vi "GetRingText.vi"(8 "error in (no error)":errorcluster, 11 "RingItem in":refnum<class "RingItem.lvclass">) -> (0 "error out":errorcluster, 2 "ring text":string, 3 "RingItem out":refnum<class "RingItem.lvclass">)   [LabVIEW 2009, in "NavScreen.lvlib" / "RingItem.lvclass"]
uses:
  RingItem.lvclass
  RingItem.lvclass/RingItem.ctl
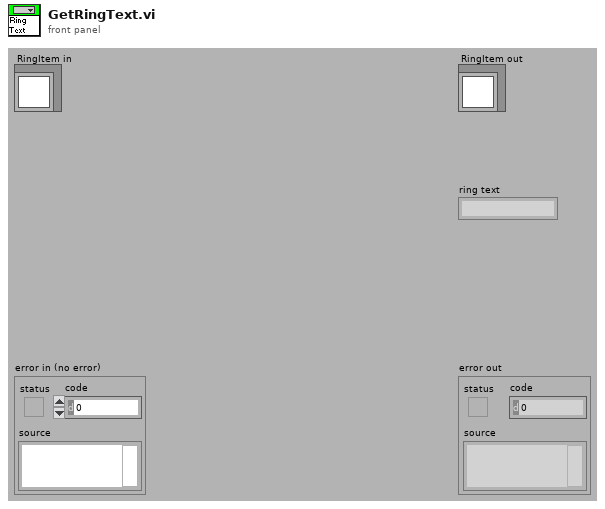
[diagram p1: front panel]
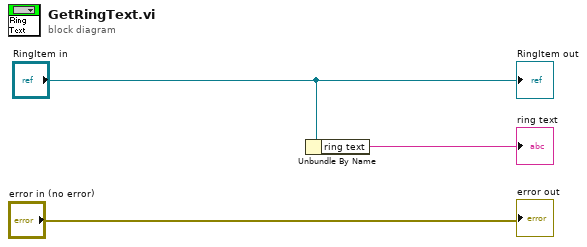
[diagram p0: block diagram]
diagram:
  n1 = Unbundle By Name("RingItem in") -> ("ring text"=→"ring text":string)
  "error out" <- "error in (no error)"
  "RingItem out" <- "RingItem in"
